vi "FestoCPX.DI.Parse.vi"(2 "Bytes DO":u16[](array[numeric]) format="%.0x") -> (10 "Raw Array":bool[](array[boolean]))   [LabVIEW 2014]
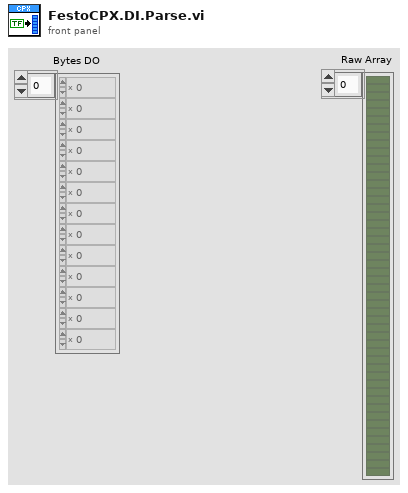
[diagram p1: front panel]
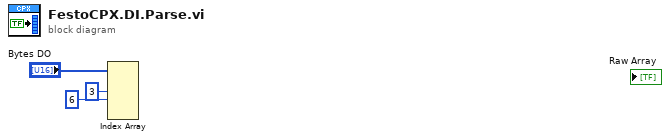
[diagram p0: block diagram]
diagram:
  n1 = Index Array(array="Bytes DO", index #2=3 ("index"), index #3=6 ("index")) -> ()  [unwired: 3 in, 5 out]
